vi "string to enum.vi"(7 "enum type":variant, 10 "error in":errorcluster, 11 "string":string) -> (2 "error out":errorcluster, 3 "enum out":variant)   [LabVIEW 2019, in "Instrument.lvclass"]
uses:
  Instrument.lvclass
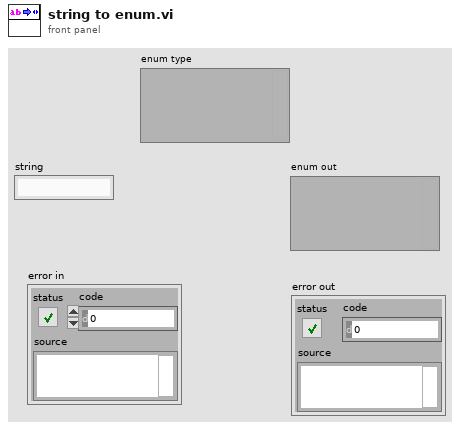
[diagram p1: front panel]
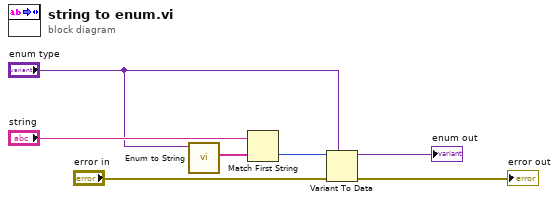
[diagram p0: block diagram]
diagram:
  n1 = call "Enum to String.vi"("Command in"="enum type") -> ("Commands out"=w7:string[])  [unwired: 9 in, 1 out]
  n2 = Match First String(2:w7, 3:"string") -> (0:w5:i32)  [unwired: 1 out]
  n3 = Variant To Data(error in="error in", type="enum type", Variant=w5) -> (data=→"enum out":variant, error out=→"error out":errorcluster)
